vi "WPI_AnalogOutputClose.vi"(8 "error in (no error)":errorcluster, 11 "AODeviceRef":T1={"DevStatus"={"status"=FALSE, "code"=0, "source"=""}, "AO Channel"=enum."Invalid"}) -> (0 "error out":errorcluster)   [LabVIEW 2017]
doc: "Closes the reference to the analog output you specify. Use this VI to close each analog output reference that you open with the Open VI.\n\nThis software is licensed. Open the labview\\readme\\WPI Robotics Library Open Source License.txt file for more information."
uses:
  <vilib>/Rock Robotics/WPI/AnalogOutput/WPI_AOChannelDevRef.ctl
  <vilib>/Rock Robotics/WPI/AnalogOutput/WPI_AnalogOutputChannel.ctl
  <vilib>/Rock Robotics/WPI/AnalogChannel/WPI_AnalogChannelChannelCacheOp.ctl
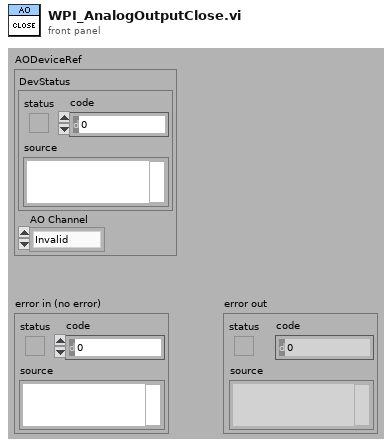
[diagram p1: front panel]
types:
  T1 = typedef "WPI_AOChannelDevRef.ctl" = cluster{"DevStatus":errorcluster, "AO Channel":T2}
  T2 = typedef "WPI_AnalogOutputChannel.ctl" = enum8{"AO MXP 0", "AO MXP 1", "Invalid"}
  T3 = typedef "WPI_AnalogChannelChannelCacheOp.ctl" = enum16{"Acquire", "Release", "Status"}
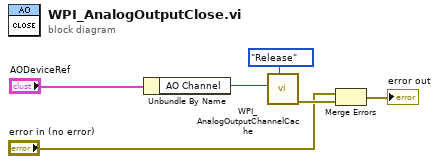
[diagram p0: block diagram]
diagram:
  n1 = Unbundle By Name("AODeviceRef") -> ("AO Channel"=w4:T2)
  n2 = call <vilib>:"WPI_AnalogOutputChannelCache.vi"("Operation"=WPI_AnalogChannelChannelCacheOp."Release", "AO Channel"=w4) -> ("error out"=w2:errorcluster)  [unwired: 7 in, 2 out]
  n3 = Merge Errors("error in (no error)", w2) -> (→"error out":errorcluster)
